vi "PATCH.vi"(8 "error in (no error)":errorcluster, 10 "url":string, 11 "Refnum in":T1) -> (0 "error out":errorcluster, 1 "body":string, 2 "headers":string, 3 "Refnum out":T1)   [LabVIEW 2018]
uses:
  <vilib>/httpClient/ClientHandle.ctl
  <vilib>/httpClient/LabVIEWHTTPClient.lvlib
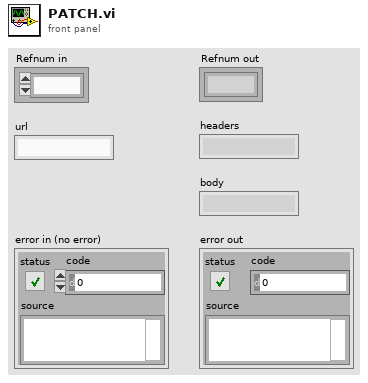
[diagram p1: front panel]
types:
  T1 = typedef "LabVIEWHTTPClient.lvlib/ClientHandle.ctl" = refnum<k1>
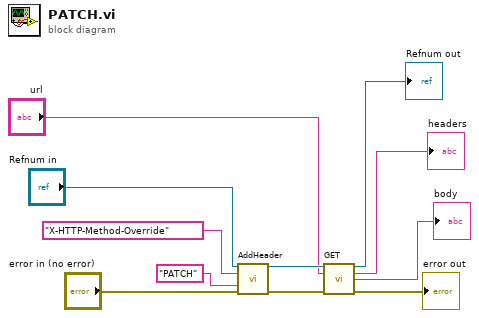
[diagram p0: block diagram]
diagram:
  n1 = call <vilib>:"AddHeader.vi"("client handle"="Refnum in", "header"="X-HTTP-Method-Override", "value"="PATCH", "error in (no error)"="error in (no error)") -> ("client handle out"=w7:T1, "error out"=w10:errorcluster)  [unwired: 10 in]
  n2 = call <vilib>:"GET.vi"("client handle"=w7, "url"="url", "error in (no error)"=w10) -> ("client handle out"=→"Refnum out":T1, "headers"=→"headers":string, "body"=→"body":string, "error out"=→"error out":errorcluster)  [unwired: 9 in]
